vi "StaticCalibration备份.vi"(0 "SENSOR":T1, 11 "error in (no error)":errorcluster caption="错误输入（无错误）") -> (4 "Vres":dbl, 6 "Angle out":dbl, 8 "Vres_FD":i32, 10 "OK？":bool, 15 "error out":errorcluster caption="错误输出")   [LabVIEW 2020]
doc: "该模板用于创建子VI。"
uses:
  Global_Variable/Global.vi
panel:
  out "T2(%)":dbl
  out "T1(%)":dbl
  out "S(%)":dbl
  out "P(%)":dbl
  out "T2ROC_1+T2ROC_2":i32
  out "T1ROC_1+T1ROC_2":i32
  out "PROC_1":i32
  out "T2ROC_1":i32
  out "T1ROC_1":i32
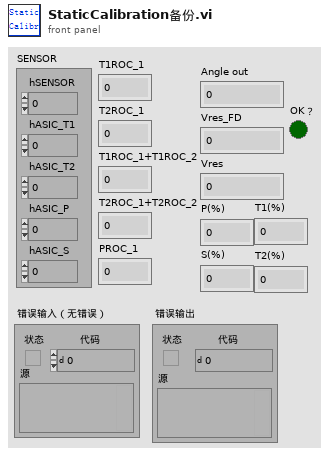
[diagram p1: front panel]
types:
  T1 = cluster{"hSENSOR":i32, "hASIC_T1":i32, "hASIC_T2":i32, "hASIC_P":i32, "hASIC_S":i32}
  T2 = cluster{"主信号":cluster{"单位":string, "下限":dbl, "上限":dbl}, "副信号":cluster{"单位":string, "下限":dbl, "上限":dbl}, "主副和":cluster{"单位":string, "下限":dbl, "上限":dbl}, "主副差":cluster{"单位":string, "下限":dbl, "上限":dbl}, "Vres":cluster{"单位":string, "下限":dbl, "上限":dbl}}
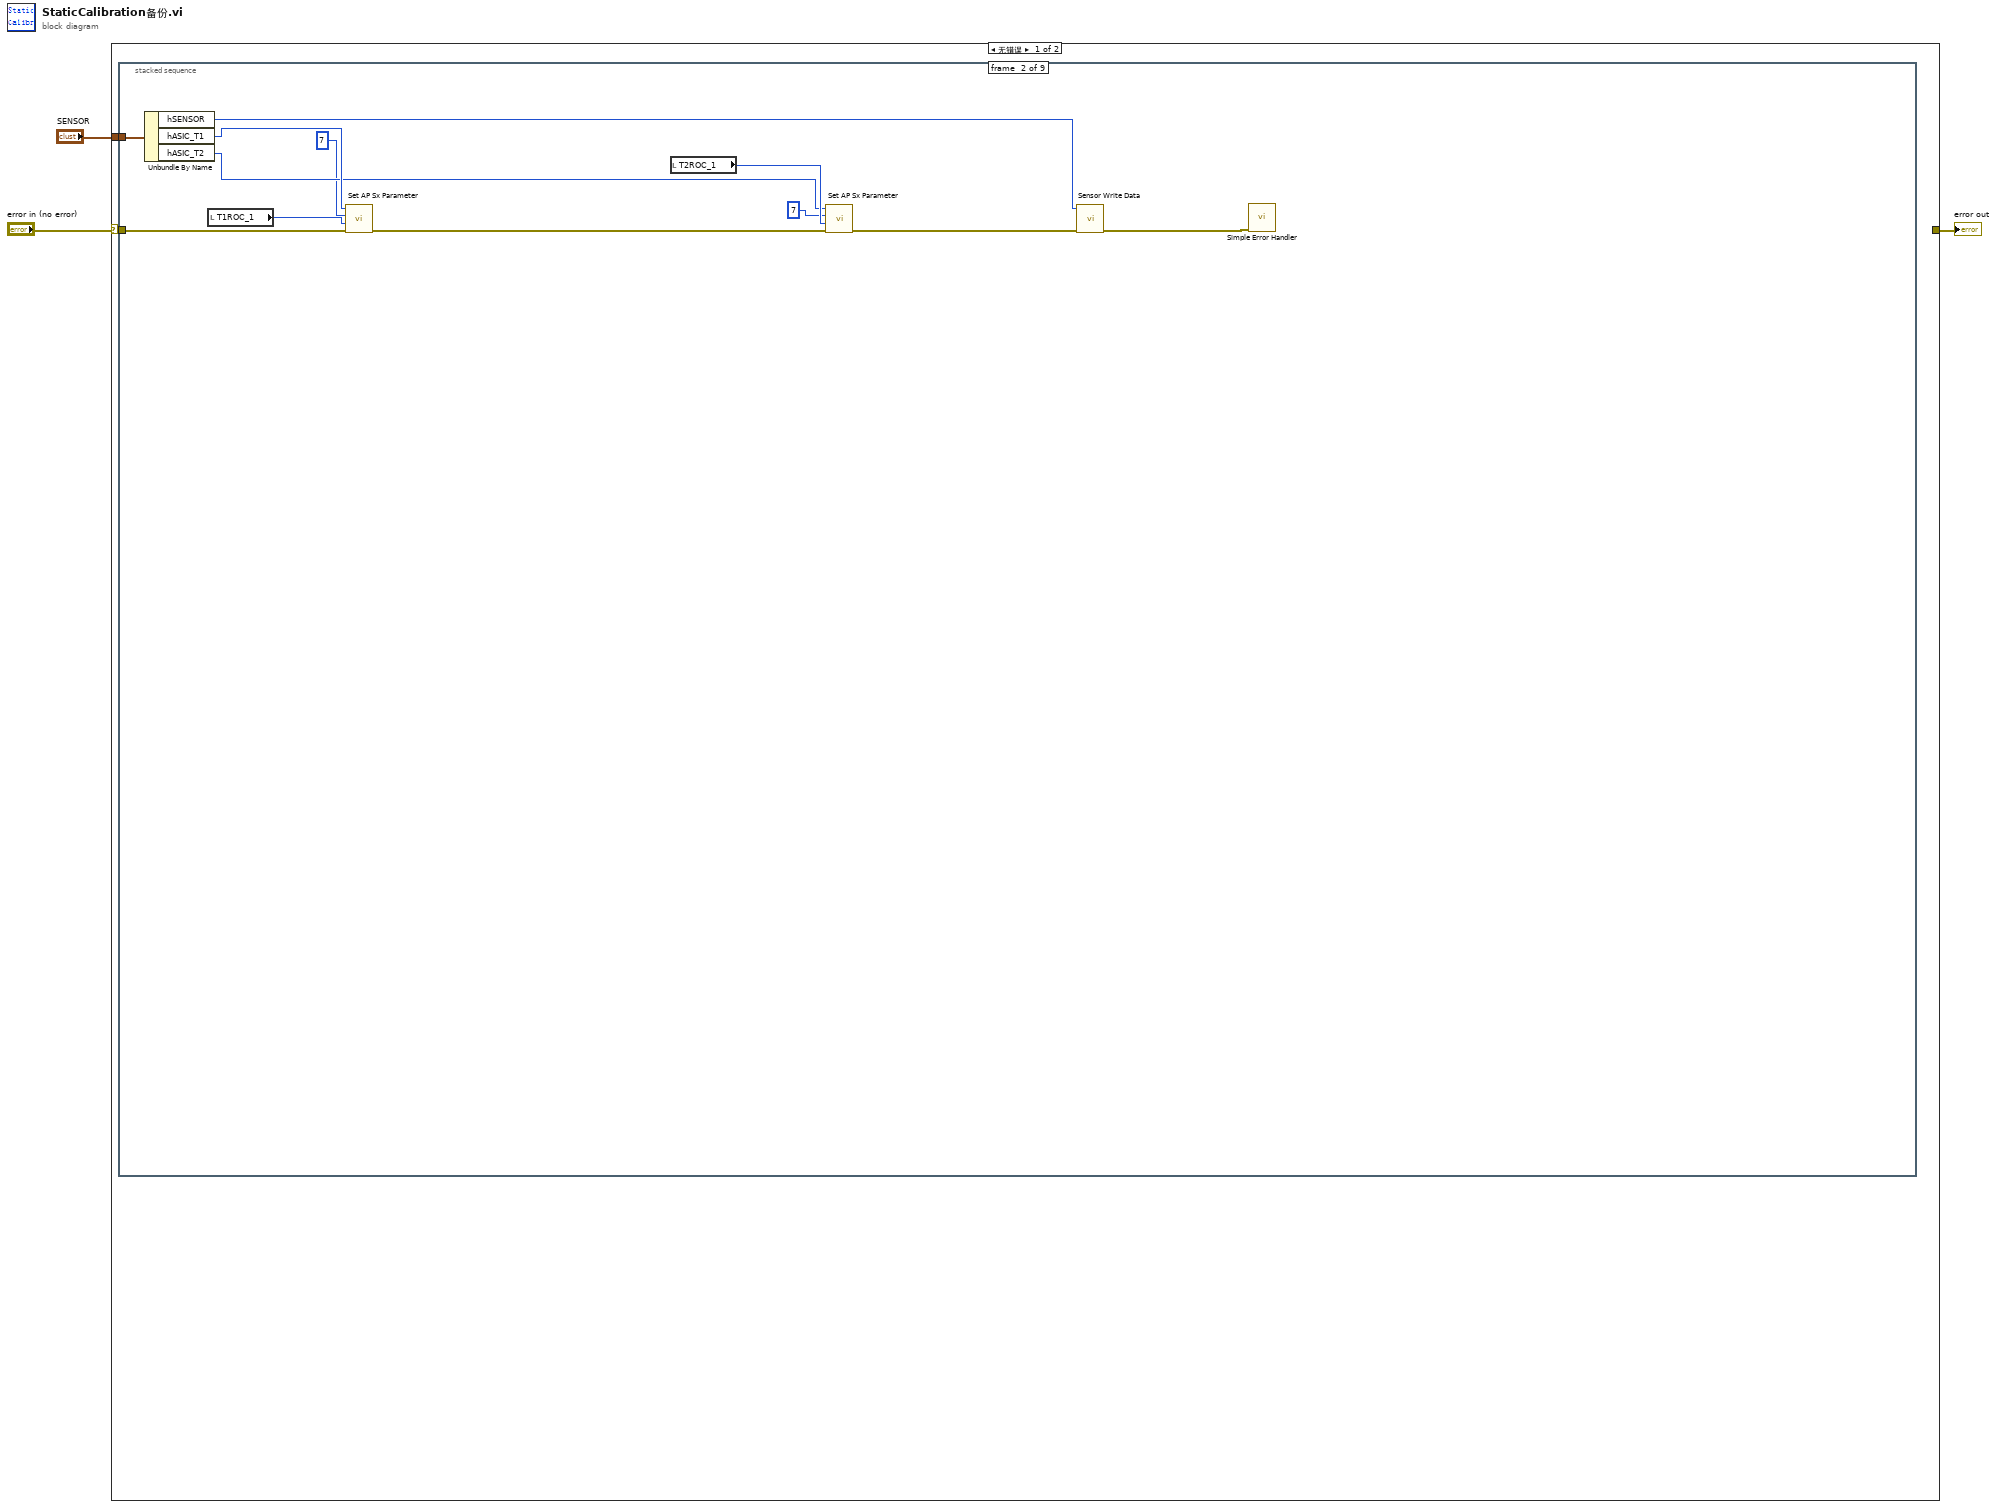
[diagram p0: block diagram]
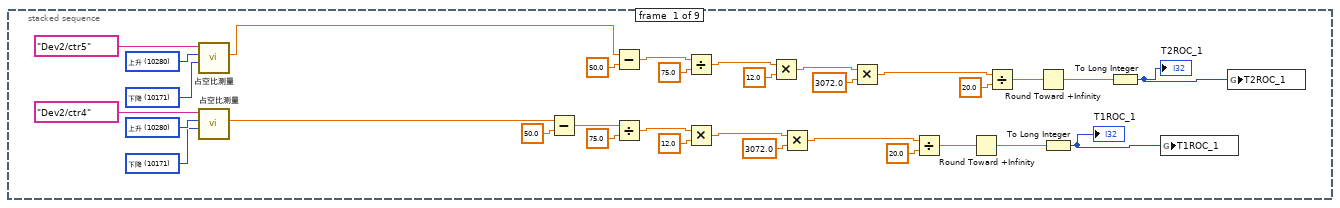
[diagram p2: hidden frame]
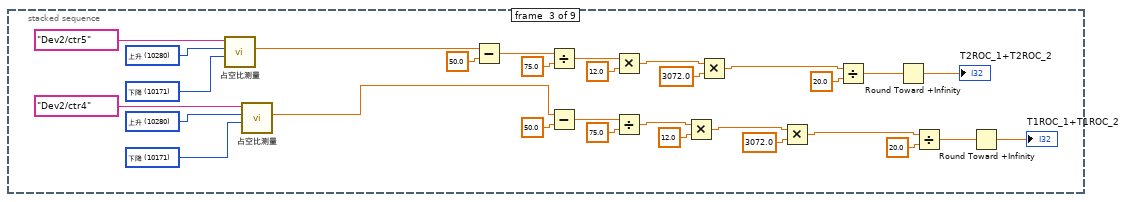
[diagram p3: hidden frame]
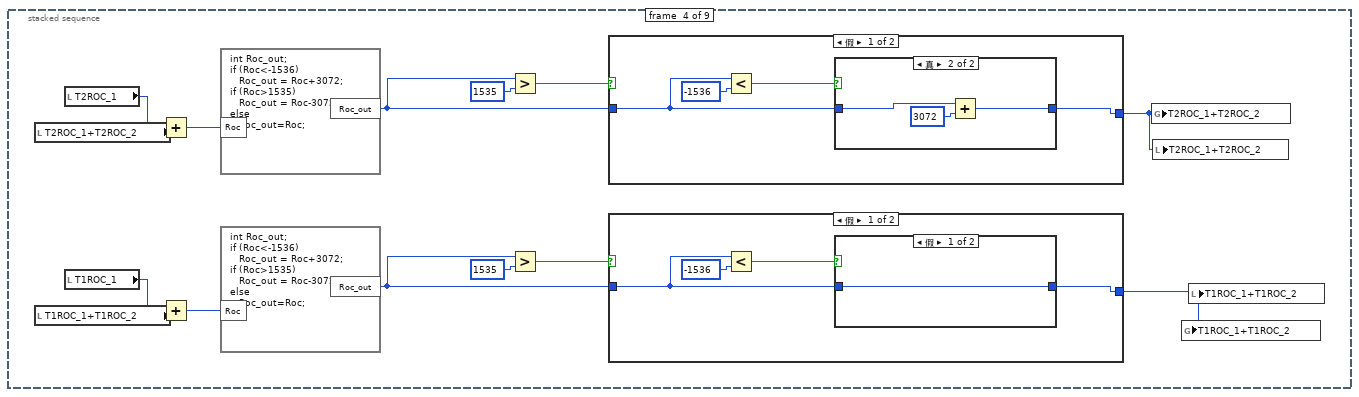
[diagram p4: hidden frame]
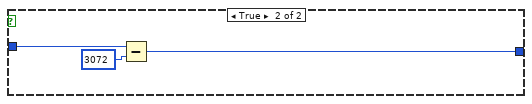
[diagram p6: hidden frame]
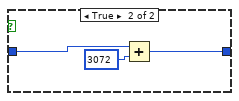
[diagram p7: hidden frame]
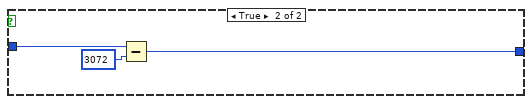
[diagram p8: hidden frame]
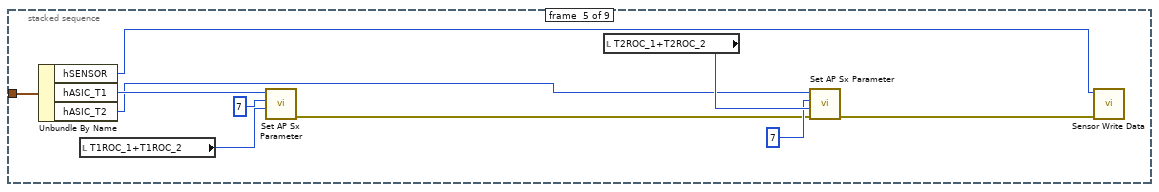
[diagram p9: hidden frame]
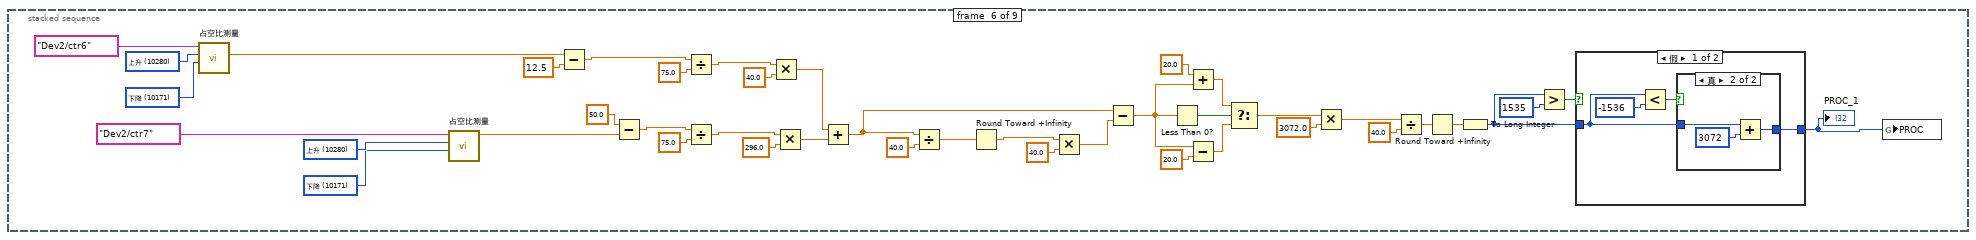
[diagram p10: hidden frame]
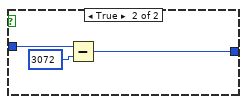
[diagram p12: hidden frame]
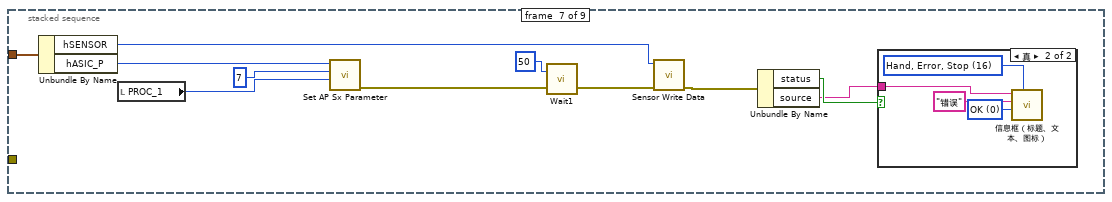
[diagram p13: hidden frame]
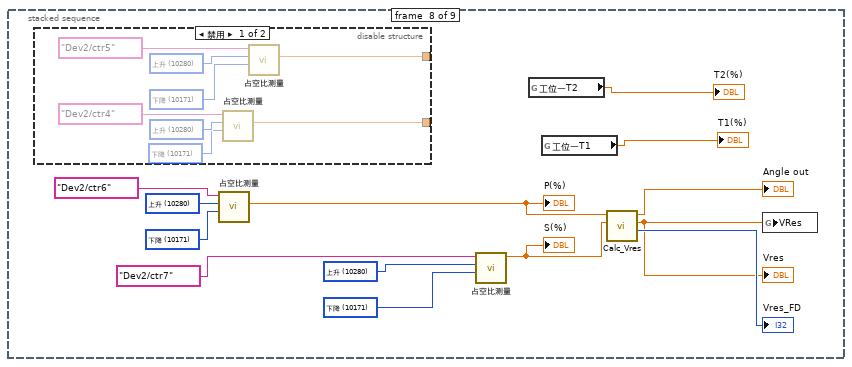
[diagram p15: hidden frame]
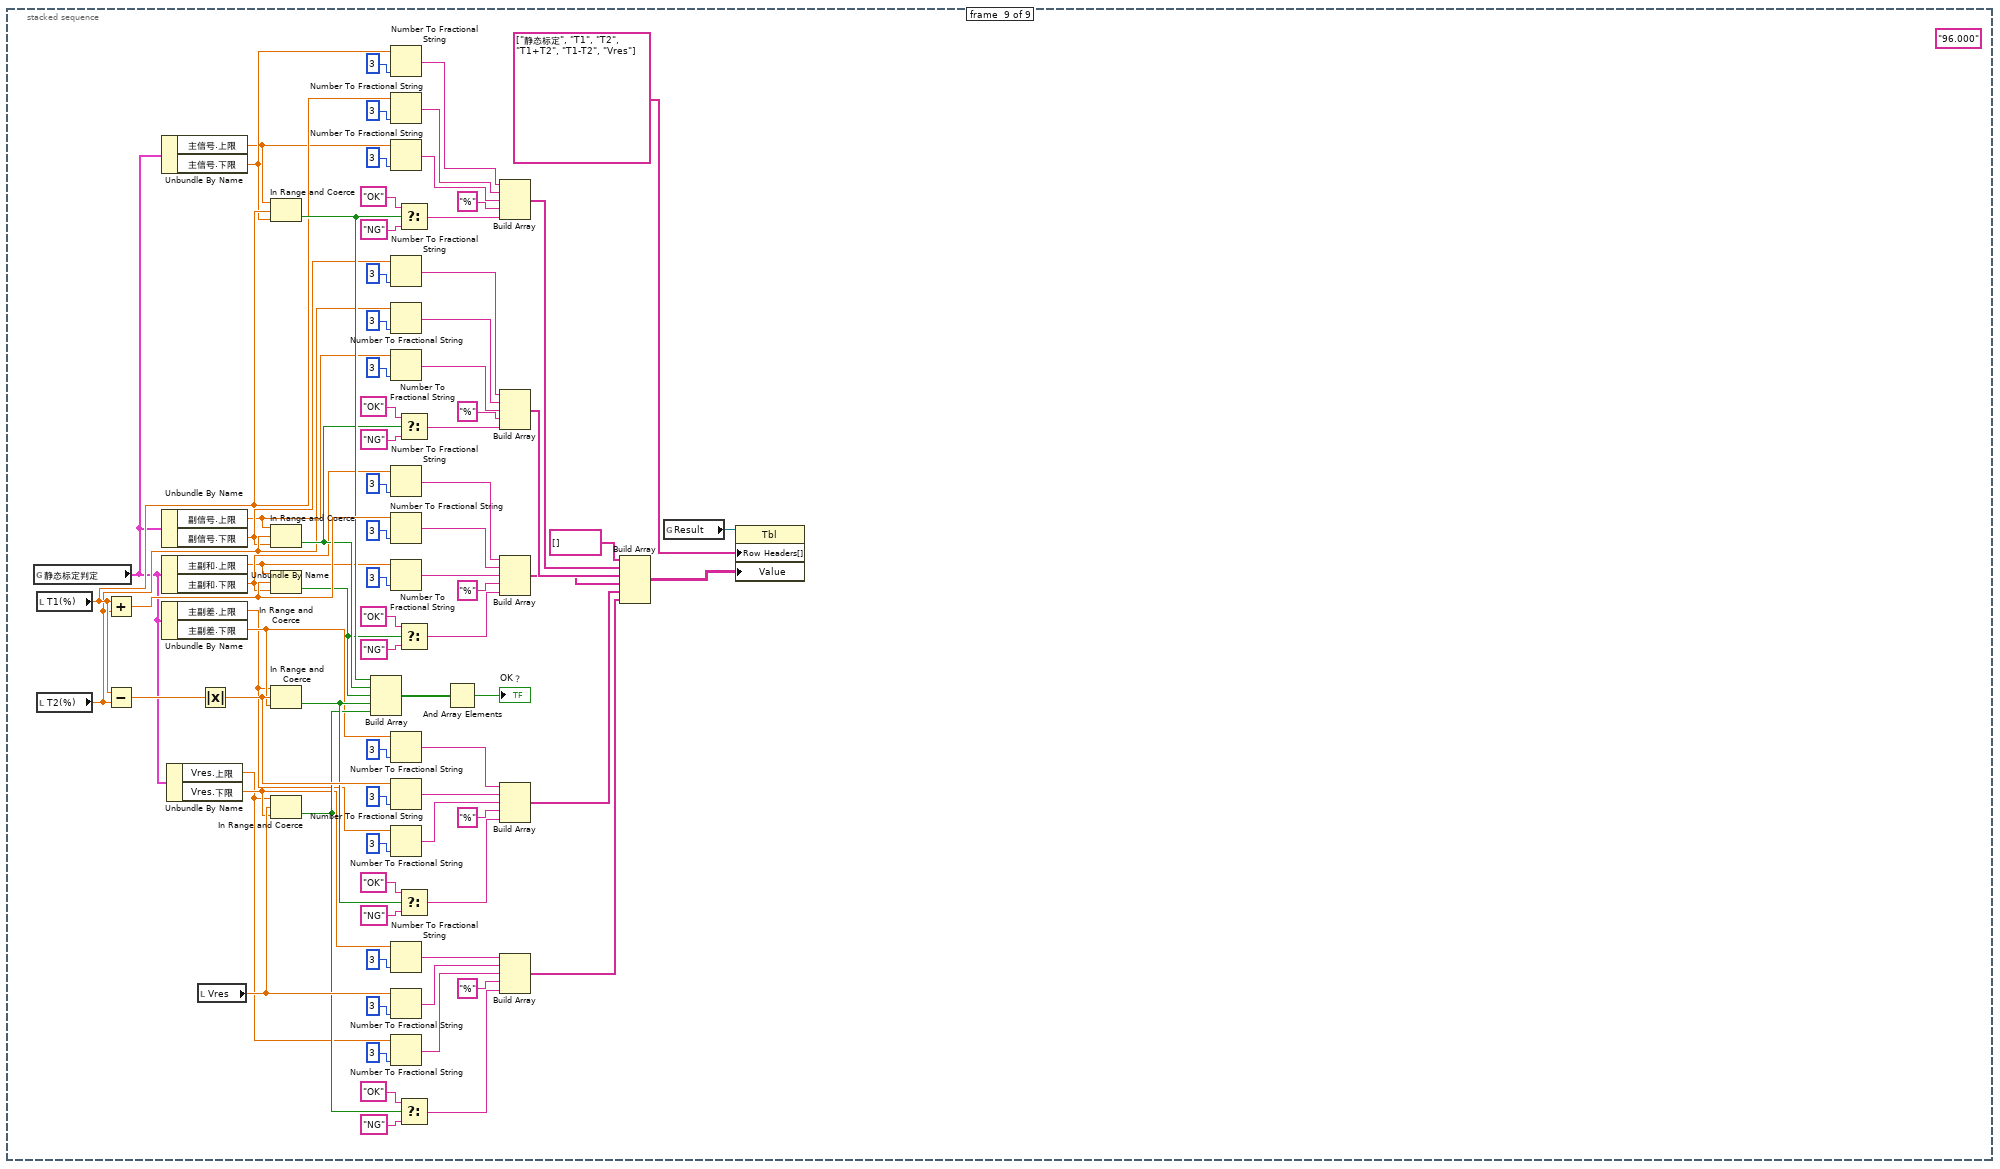
[diagram p17: hidden frame]
diagram:
  n1 = case shown="无错误" "error in (no error)" {
    selector: "error in (no error)" -> [w4 w298]
    tunnel: [_ w298] -> w2
    tunnel: "SENSOR" -> [w5 _]
    frame No Error {
      n2 = stacked-sequence {
        tunnel: w5 -> [_ w47 _ _ w124 _ w184 _ _]
        tunnel: w4 -> [_ w39 _ _ _ _ _ _ _]
        frame #0 {
          w6 = 10171 items=["上升"=10280, "下降"=10171] ("starting edge2")
          w7 = 10280 items=["上升"=10280, "下降"=10171] ("starting edge1")
          w8 = 10171 items=["上升"=10280, "下降"=10171] ("starting edge2")
          w9 = 10280 items=["上升"=10280, "下降"=10171] ("starting edge1")
          n3 = call "占空比测量.vi"("计数器"=tag "Dev2/ctr5" ("counter"), "starting edge1"=w7, "starting edge2"=w6) -> ("占空比2(%)"=w10:dbl)  [unwired: 4 in, 3 out]
          n4 = call "占空比测量.vi"("计数器"=tag "Dev2/ctr4" ("counter"), "starting edge1"=w9, "starting edge2"=w8) -> ("占空比2(%)"=w13:dbl)  [unwired: 4 in, 3 out]
          n5 = Subtract(x=w13, y=50.0) -> (x-y=w36:dbl)
          n6 = Subtract(x=w10, y=50.0) -> (x-y=w21:dbl)
          n7 = Divide(x=w36, y=75.0) -> (x/y=w34:dbl)
          n8 = Divide(x=w21, y=75.0) -> (x/y=w23:dbl)
          n9 = Multiply(x=w34, y=12.0) -> (x*y=w32:dbl)
          n10 = Multiply(x=w23, y=12.0) -> (x*y=w25:dbl)
          n11 = Multiply(x=w32, y=3072.0) -> (x*y=w30:dbl)
          n12 = Multiply(x=w25, y=3072.0) -> (x*y=w27:dbl)
          n13 = Divide(x=w30, y=20.0) -> (x/y=w17:dbl)
          n14 = Round Toward +Infinity(x=w17) -> (ceil(x): smallest int >= x=w15:dbl)
          n15 = Divide(x=w27, y=20.0) -> (x/y=w16:dbl)
          n16 = Round Toward +Infinity(x=w16) -> (ceil(x): smallest int >= x=w14:dbl)
          n17 = To Long Integer(number=w15) -> (32bit integer=w11:i32)
          "T1ROC_1" <- w11
          n18 = To Long Integer(number=w14) -> (32bit integer=w12:i32)
          "T2ROC_1" <- w12
          n19 = global write "Global.vi" "T1ROC_1"(w11) -> ()
          n20 = global write "Global.vi" "T2ROC_1"(w12) -> ()
        }
        frame #1 {
          n21 = Unbundle By Name(w47) -> ("hSENSOR"=w44:i32, "hASIC_T1"=w46:i32, "hASIC_T2"=w45:i32)
          n22 = local read "T1ROC_1"() -> (w48:i32)
          n23 = call "Set AP Sx Parameter.vi"("error in (no error)"=w39, "para2"=w48, "asicBitsName"=7, "asicHandle"=w46) -> ("error out"=w41:errorcluster)  [unwired: 6 in, 1 out]
          n24 = local read "T2ROC_1"() -> (w49:i32)
          n25 = call "Set AP Sx Parameter.vi"("error in (no error)"=w41, "para2"=w49, "asicBitsName"=7, "asicHandle"=w45) -> ("error out"=w40:errorcluster)  [unwired: 6 in, 1 out]
          n26 = call "Sensor Write Data.vi"("error in (no error)"=w40, "sensorHandle"=w44) -> ("error out"=w38:errorcluster)  [unwired: 8 in, 1 out]
          n27 = call <vilib>:"Simple Error Handler.vi"("error in (no error)"=w38) -> ()  [unwired: 4 in, 5 out]
        }
        frame #2 {
          w50 = 10171 items=["上升"=10280, "下降"=10171] ("starting edge2")
          w51 = 10280 items=["上升"=10280, "下降"=10171] ("starting edge1")
          w52 = 10171 items=["上升"=10280, "下降"=10171] ("starting edge2")
          w53 = 10280 items=["上升"=10280, "下降"=10171] ("starting edge1")
          n28 = call "占空比测量.vi"("计数器"=tag "Dev2/ctr5", "starting edge1"=w51, "starting edge2"=w50) -> ("占空比2(%)"=w57:dbl)  [unwired: 4 in, 3 out]
          n29 = call "占空比测量.vi"("计数器"=tag "Dev2/ctr4", "starting edge1"=w53, "starting edge2"=w52) -> ("占空比2(%)"=w54:dbl)  [unwired: 4 in, 3 out]
          n30 = Subtract(x=w57, y=50.0) -> (x-y=w79:dbl)
          n31 = Divide(x=w79, y=75.0) -> (x/y=w78:dbl)
          n32 = Subtract(x=w54, y=50.0) -> (x-y=w72:dbl)
          n33 = Multiply(x=w78, y=12.0) -> (x*y=w77:dbl)
          n34 = Divide(x=w72, y=75.0) -> (x/y=w73:dbl)
          n35 = Multiply(x=w73, y=12.0) -> (x*y=w74:dbl)
          n36 = Multiply(x=w77, y=3072.0) -> (x*y=w76:dbl)
          n37 = Multiply(x=w74, y=3072.0) -> (x*y=w75:dbl)
          n38 = Divide(x=w76, y=20.0) -> (x/y=w70:dbl)
          n39 = Round Toward +Infinity(x=w70) -> (ceil(x): smallest int >= x=→"T2ROC_1+T2ROC_2":dbl)
          n40 = Divide(x=w75, y=20.0) -> (x/y=w71:dbl)
          n41 = Round Toward +Infinity(x=w71) -> (ceil(x): smallest int >= x=→"T1ROC_1+T1ROC_2":dbl)
        }
        frame #3 {
          n42 = local read "T2ROC_1+T2ROC_2"() -> (w82:i32)
          n43 = local read "T1ROC_1+T1ROC_2"() -> (w83:i32)
          n44 = local read "T2ROC_1"() -> (w90:i32)
          n45 = local read "T1ROC_1"() -> (w91:i32)
          n46 = Add(x=w90, y=w82) -> (x+y=w92:i32)
          n47 = Add(x=w91, y=w83) -> (x+y=w93:i32)
          n48 = formula code="int Roc_out;\nif (Roc<-1536)\n   Roc_out = Roc+3072;\nif (Roc>1535)\n   Roc_out = Roc-3072;\nelse\n   Roc_out=Roc;"("Roc"=w92) -> ("Roc_out"=w84:i32)
          n49 = formula code="int Roc_out;\nif (Roc<-1536)\n   Roc_out = Roc+3072;\nif (Roc>1535)\n   Roc_out = Roc-3072;\nelse\n   Roc_out=Roc;"("Roc"=w93) -> ("Roc_out"=w87:i32)
          n50 = Greater?(x=w84, y=1535) -> (0:w85:bool)
          n51 = Greater?(x=w87, y=1535) -> (0:w88:bool)
          n52 = case shown="假" w85 {
            tunnel: w84 -> [w95 w103]
            tunnel: [w94 w102] -> w80
            frame False {
              n53 = Less?(x=w95, y=-1536) -> (x < y?=w96:bool)
              n54 = case shown="真" w96 {
                tunnel: w95 -> [w98 w101]
                tunnel: [w98 w99] -> w94
                frame False {
                }
                frame True {
                  n55 = Add(x=w101, y=3072) -> (x+y=w99:i32)
                }
              }
            }
            frame True {
              n56 = Subtract(x=w103, y=3072) -> (x-y=w102:i32)
            }
          }
          n57 = case shown="假" w88 {
            tunnel: w87 -> [w106 w114]
            tunnel: [w105 w113] -> w81
            frame False {
              n58 = Less?(x=w106, y=-1536) -> (x < y?=w107:bool)
              n59 = case shown="假" w107 {
                tunnel: w106 -> [w109 w112]
                tunnel: [w109 w110] -> w105
                frame False {
                }
                frame True {
                  n60 = Add(x=w112, y=3072) -> (x+y=w110:i32)
                }
              }
            }
            frame True {
              n61 = Subtract(x=w114, y=3072) -> (x-y=w113:i32)
            }
          }
          n62 = global write "Global.vi" "T2ROC_1+T2ROC_2"(w80) -> ()
          n63 = local write "T2ROC_1+T2ROC_2"(w80) -> ()
          n64 = global write "Global.vi" "T1ROC_1+T1ROC_2"(w81) -> ()
          n65 = local write "T1ROC_1+T1ROC_2"(w81) -> ()
        }
        frame #4 {
          n66 = Unbundle By Name(w124) -> ("hSENSOR"=w121:i32, "hASIC_T1"=w123:i32, "hASIC_T2"=w122:i32)
          n67 = local read "T1ROC_1+T1ROC_2"() -> (w120:i32)
          n68 = call "Set AP Sx Parameter.vi"("para2"=w120, "asicBitsName"=7, "asicHandle"=w123) -> ("error out"=w117:errorcluster)  [unwired: 7 in, 1 out]
          n69 = local read "T2ROC_1+T2ROC_2"() -> (w125:i32)
          n70 = call "Set AP Sx Parameter.vi"("error in (no error)"=w117, "para2"=w125, "asicBitsName"=7, "asicHandle"=w122) -> ("error out"=w116:errorcluster)  [unwired: 6 in, 1 out]
          n71 = call "Sensor Write Data.vi"("error in (no error)"=w116, "sensorHandle"=w121) -> ()  [unwired: 8 in, 2 out]
        }
        frame #5 {
          w126 = 10171 items=["上升"=10280, "下降"=10171] ("starting edge2")
          w127 = 10280 items=["上升"=10280, "下降"=10171] ("starting edge1")
          w128 = 10171 items=["上升"=10280, "下降"=10171] ("starting edge2")
          w129 = 10280 items=["上升"=10280, "下降"=10171] ("starting edge1")
          n72 = call "占空比测量.vi"("计数器"=tag "Dev2/ctr6", "starting edge1"=w129, "starting edge2"=w128) -> ("占空比2(%)"=w134:dbl)  [unwired: 4 in, 3 out]
          n73 = call "占空比测量.vi"("计数器"=tag "Dev2/ctr7", "starting edge1"=w127, "starting edge2"=w126) -> ("占空比(%)"=w133:dbl)  [unwired: 4 in, 3 out]
          n74 = Subtract(x=w134, y=12.5) -> (x-y=w166:dbl)
          n75 = Subtract(x=50.0, y=w133) -> (x-y=w160:dbl)
          n76 = Divide(x=w166, y=75.0) -> (x/y=w164:dbl)
          n77 = Divide(x=w160, y=75.0) -> (x/y=w158:dbl)
          n78 = Multiply(x=w164, y=40.0) -> (x*y=w162:dbl)
          n79 = Multiply(x=w158, y=296.0) -> (x*y=w156:dbl)
          n80 = Add(x=w162, y=w156) -> (x+y=w150:dbl)
          n81 = Divide(x=w150, y=40.0) -> (x/y=w154:dbl)
          n82 = Round Toward +Infinity(x=w154) -> (ceil(x): smallest int >= x=w152:dbl)
          n83 = Multiply(x=w152, y=40.0) -> (x*y=w151:dbl)
          n84 = Subtract(x=w150, y=w151) -> (x-y=w146:dbl)
          n85 = Less Than 0?(x=w146) -> (x < 0?=w145:bool)
          n86 = Add(x=20.0, y=w146) -> (x+y=w148:dbl)
          n87 = Subtract(x=w146, y=20.0 ("x")) -> (x-y=w144:dbl)
          n88 = Select(t=w148, s=w145, f=w144) -> (s? t:f=w143:dbl)
          n89 = Multiply(x=w143, y=3072.0) -> (x*y=w141:dbl)
          n90 = Divide(x=w141, y=40.0) -> (x/y=w136:dbl)
          n91 = Round Toward +Infinity(x=w136) -> (ceil(x): smallest int >= x=w135:dbl)
          n92 = To Long Integer(number=w135) -> (32bit integer=w139:i32)
          n93 = Greater?(x=w139, y=1535) -> (0:w137:bool)
          n94 = case shown="假" w137 {
            tunnel: w139 -> [w169 w177]
            tunnel: [w168 w176] -> w130
            frame False {
              n95 = Less?(x=w169, y=-1536) -> (x < y?=w170:bool)
              n96 = case shown="真" w170 {
                tunnel: w169 -> [w172 w175]
                tunnel: [w172 w173] -> w168
                frame False {
                }
                frame True {
                  n97 = Add(x=w175, y=3072) -> (x+y=w173:i32)
                }
              }
            }
            frame True {
              n98 = Subtract(x=w177, y=3072) -> (x-y=w176:i32)
            }
          }
          "PROC_1" <- w130
          n99 = global write "Global.vi" "PROC"(w130) -> ()
        }
        frame #6 {
          n100 = Unbundle By Name(w184) -> ("hSENSOR"=w183:i32, "hASIC_P"=w182:i32)
          n101 = local read "PROC_1"() -> (w187:i32)
          n102 = call "Set AP Sx Parameter.vi"("para2"=w187, "asicBitsName"=7, "asicHandle"=w182) -> ("error out"=w189:errorcluster)  [unwired: 7 in, 1 out]
          n103 = call "Wait1.vi"("error in (no error)"=w189, "Wait（150ms）"=u32 50) -> ("error out"=w188:errorcluster)  [unwired: 1 in]
          n104 = call "Sensor Write Data.vi"("error in (no error)"=w188, "sensorHandle"=w183) -> ("error out"=w181:errorcluster)  [unwired: 8 in, 1 out]
          n105 = Unbundle By Name(w181) -> ("status"=w180:bool, "source"=w179:string)
          n106 = case shown="真" w180 {
            tunnel: w179 -> [_ w190]
            frame False {
            }
            frame True {
              w191 = 16 items=["None"=0, "Hand, Error, Stop"=16, "Question"=32, "Exclamation, Warning"=48, "Asterisk, Information"=64] ("icon")
              w192 = 0 items=["OK", "OKCancel", "AbortRetryIgnore", "YesNoCancel", "YesNo", "RetryCancel"] ("buttons")
              n107 = call "信息框（标题、文本、图标）.vi"("icon"=w191, "buttons"=w192, "caption"="错误", "text"=w190) -> ()  [unwired: 6 in, 2 out]
            }
          }
        }
        frame #7 {
          w196 = 10171 items=["上升"=10280, "下降"=10171] ("starting edge2")
          w197 = 10280 items=["上升"=10280, "下降"=10171] ("starting edge1")
          w198 = 10171 items=["上升"=10280, "下降"=10171] ("starting edge2")
          w199 = 10280 items=["上升"=10280, "下降"=10171] ("starting edge1")
          n108 = disable-structure shown="禁用" {
            disable-tunnel: [w212 _] -> _
            disable-tunnel: [w211 _] -> _
            frame Disabled {
              w207 = 10171 items=["上升"=10280, "下降"=10171] ("starting edge2")
              w208 = 10280 items=["上升"=10280, "下降"=10171] ("starting edge1")
              w209 = 10171 items=["上升"=10280, "下降"=10171] ("starting edge2")
              w210 = 10280 items=["上升"=10280, "下降"=10171] ("starting edge1")
              n109 = call "占空比测量.vi"("计数器"=tag "Dev2/ctr4", "starting edge1"=w210, "starting edge2"=w209) -> ("占空比2(%)"=w212:dbl)  [unwired: 4 in, 3 out]
              n110 = call "占空比测量.vi"("计数器"=tag "Dev2/ctr5", "starting edge1"=w208, "starting edge2"=w207) -> ("占空比2(%)"=w211:dbl)  [unwired: 4 in, 3 out]
            }
            frame Enabled {
            }
          }
          n111 = call "占空比测量.vi"("计数器"=tag "Dev2/ctr6", "starting edge1"=w199, "starting edge2"=w198) -> ("占空比2(%)"=w204:dbl)  [unwired: 4 in, 3 out]
          "P(%)" <- w204
          n112 = call "占空比测量.vi"("计数器"=tag "Dev2/ctr7", "starting edge1"=w197, "starting edge2"=w196) -> ("占空比(%)"=w203:dbl)  [unwired: 4 in, 3 out]
          "S(%)" <- w203
          n113 = global read "Global.vi" "工位一T2"() -> (→"T2(%)":dbl)
          n114 = global read "Global.vi" "工位一T1"() -> (→"T1(%)":dbl)
          n115 = call "Calc_Vres.vi"("S_Data in"=w203, "P_Data in"=w204) -> ("Vres_FD"=→"Vres_FD":i32, "Vres"=w200:dbl, "Angle out"=→"Angle out":dbl)  [unwired: 7 in]
          "Vres" <- w200
          n116 = global write "Global.vi" "VRes"(w200) -> ()
        }
        frame #8 {
          (unwired) "96.000"
          n117 = global read "Global.vi" "静态标定判定"() -> (w249:T2)
          n118 = local read "T1(%)"() -> (w252:dbl)
          n119 = local read "T2(%)"() -> (w251:dbl)
          n120 = Add(x=w252, y=w251) -> (x+y=w288:dbl)
          n121 = Subtract(x=w252, y=w251) -> (x-y=w255:dbl)
          n122 = Unbundle By Name(w249) -> ("主信号.上限"=w234:dbl, "主信号.下限"=w236:dbl)
          n123 = Unbundle By Name(w249) -> ("副信号.上限"=w231:dbl, "副信号.下限"=w232:dbl)
          n124 = Unbundle By Name(w249) -> ("主副和.上限"=w227:dbl, "主副和.下限"=w228:dbl)
          n125 = Unbundle By Name(w249) -> ("主副差.上限"=w225:dbl, "主副差.下限"=w226:dbl)
          n126 = Unbundle By Name(w249) -> ("Vres.上限"=w223:dbl, "Vres.下限"=w224:dbl)
          n127 = local read "Vres"() -> (w292:dbl)
          n128 = Absolute Value(x=w255) -> (abs(x)=w250:dbl)
          n129 = In Range and Coerce(upper limit=w234, x=w252, lower limit=w236) -> (In Range?=w265:bool)  [unwired: 1 out]
          n130 = In Range and Coerce(upper limit=w231, x=w251, lower limit=w232) -> (In Range?=w264:bool)  [unwired: 1 out]
          n131 = In Range and Coerce(upper limit=w227, x=w288, lower limit=w228) -> (In Range?=w263:bool)  [unwired: 1 out]
          n132 = In Range and Coerce(upper limit=w225, x=w250, lower limit=w226) -> (In Range?=w248:bool)  [unwired: 1 out]
          n133 = In Range and Coerce(upper limit=w223, x=w292, lower limit=w224) -> (In Range?=w247:bool)  [unwired: 1 out]
          n134 = Build Array(w265, w264, w263, w248, w247) -> (w262:bool[])
          n135 = Number To Fractional String(number=w236, precision (6)=i16 3 ("精度(6)")) -> (F-format string=w235:string)  [unwired: 2 in]
          n136 = Number To Fractional String(number=w252, precision (6)=i16 3 ("精度(6)")) -> (F-format string=w287:string)  [unwired: 2 in]
          n137 = Number To Fractional String(number=w234, precision (6)=i16 3 ("精度(6)")) -> (F-format string=w233:string)  [unwired: 2 in]
          n138 = Number To Fractional String(number=w232, precision (6)=i16 3 ("精度(6)")) -> (F-format string=w230:string)  [unwired: 2 in]
          n139 = Number To Fractional String(number=w251, precision (6)=i16 3 ("精度(6)")) -> (F-format string=w281:string)  [unwired: 2 in]
          n140 = Number To Fractional String(number=w231, precision (6)=i16 3 ("精度(6)")) -> (F-format string=w229:string)  [unwired: 2 in]
          n141 = Number To Fractional String(number=w228, precision (6)=i16 3 ("精度(6)")) -> (F-format string=w222:string)  [unwired: 2 in]
          n142 = Number To Fractional String(number=w288, precision (6)=i16 3 ("精度(6)")) -> (F-format string=w275:string)  [unwired: 2 in]
          n143 = Number To Fractional String(number=w227, precision (6)=i16 3 ("精度(6)")) -> (F-format string=w221:string)  [unwired: 2 in]
          n144 = Number To Fractional String(number=w226, precision (6)=i16 3 ("精度(6)")) -> (F-format string=w220:string)  [unwired: 2 in]
          n145 = Number To Fractional String(number=w250, precision (6)=i16 3 ("精度(6)")) -> (F-format string=w260:string)  [unwired: 2 in]
          n146 = Number To Fractional String(number=w225, precision (6)=i16 3 ("精度(6)")) -> (F-format string=w219:string)  [unwired: 2 in]
          n147 = Number To Fractional String(number=w224, precision (6)=i16 3 ("精度(6)")) -> (F-format string=w218:string)  [unwired: 2 in]
          n148 = Number To Fractional String(number=w292, precision (6)=i16 3 ("精度(6)")) -> (F-format string=w271:string)  [unwired: 2 in]
          n149 = Number To Fractional String(number=w223, precision (6)=i16 3 ("精度(6)")) -> (F-format string=w217:string)  [unwired: 2 in]
          n150 = Select(t="OK", s=w265, f="NG") -> (s? t:f=w285:string)
          n151 = Select(t="OK", s=w264, f="NG") -> (s? t:f=w284:string)
          n152 = Select(t="OK", s=w263, f="NG") -> (s? t:f=w276:string)
          n153 = Select(t="OK", s=w248, f="NG") -> (s? t:f=w259:string)
          n154 = Select(t="OK", s=w247, f="NG") -> (s? t:f=w274:string)
          n155 = And Array Elements(Boolean array=w262) -> (logical AND=→"OK？":bool)
          n156 = Build Array(w235, w287, w233, "%", w285) -> (w216:string[])
          n157 = Build Array(w230, w281, w229, "%", w284) -> (w269:string[])
          n158 = Build Array(w222, w275, w221, "%", w276) -> (w268:string[])
          n159 = Build Array(w220, w260, w219, "%", w259) -> (w253:string[])
          n160 = Build Array(w218, w271, w217, "%", w274) -> (w267:string[])
          n161 = Build Array(string[] [] ("元素"), w216, w269, w268, w253, w267) -> (w266:string[][])
          n162 = global read "Global.vi" "Result"() -> (w297:refnum<vi>)
          n163 = property class="Tbl"(reference=w297, "Row Headers[]"=string[] ["静态标定", "T1", "T2", "T1+T2", "T1-T2", "Vres"] ("行首字符串[]"), "Value"=w266) -> ()  [unwired: 1 in, 2 out]
        }
      }
    }
    frame Error {
    }
  }
  "error out" <- w2
